vi "dfd_DA Index Genenration.vi"(9 "load":bool=TRUE, 10 "shift enable":bool=TRUE, 11 "shift in":bool[](array[boolean])=[FALSE, FALSE, FALSE, FALSE, FALSE, FALSE, FALSE, FALSE]) -> (3 "idx":bool[](array[boolean]))   [LabVIEW 2017]
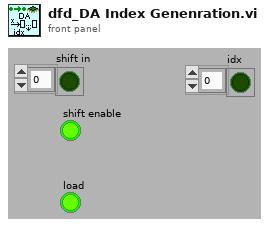
[diagram p1: front panel]
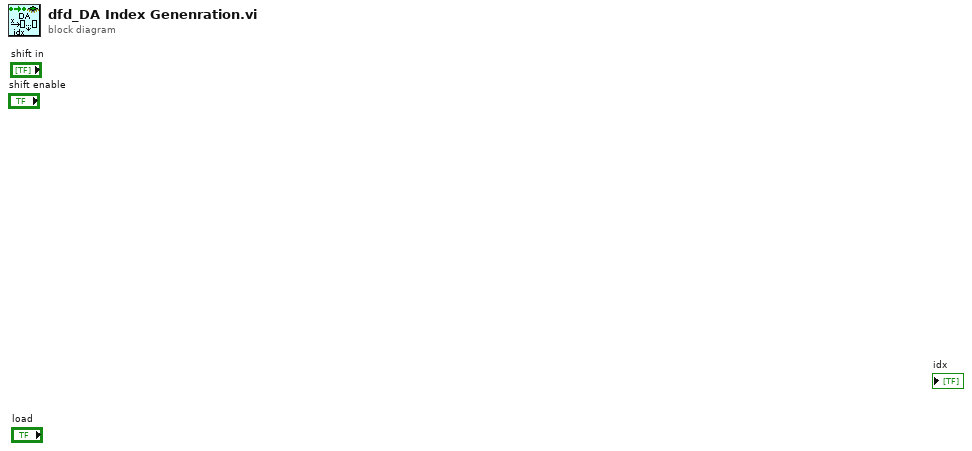
[diagram p0: block diagram]
diagram:
